vi "_Remove Capabilities.vi"(8 "error in (no error)":errorcluster, 10 "Capabilities":string[](array[string]), 11 "NodeDiscovery in":refnum<class "NodeDiscovery.lvclass">) -> (0 "error out":errorcluster, 3 "NodeDiscovery out":refnum<class "NodeDiscovery.lvclass">)   [LabVIEW 2020, in "Vecto.lvlib" / "NodeDiscovery.lvclass"]
uses:
  NodeDiscovery.lvclass
  NodeDiscovery.lvclass/NodeDiscovery.ctl
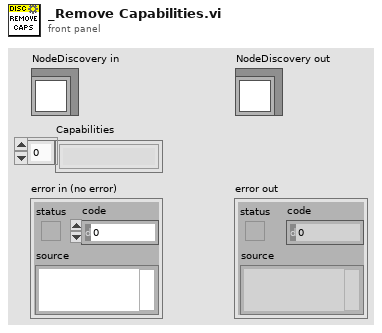
[diagram p1: front panel]
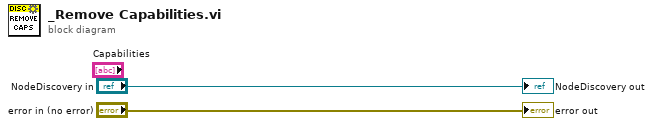
[diagram p0: block diagram]
diagram:
  "error out" <- "error in (no error)"
  "NodeDiscovery out" <- "NodeDiscovery in"
